vi "数据查询筛选.vi"() -> (2 "分钟小时":string(combo)="实时数据", 3 "工作类型":string(combo)="全部数据")   [LabVIEW 2016, in "斯坦道CODMn.lvlib"]
panel:
  in  "布尔":bool
  in  "数据类型 2":string(combo)="实时数据"
  in  "数据类型":string(combo)="全部数据"
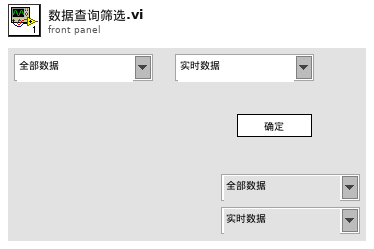
[diagram p1: front panel]
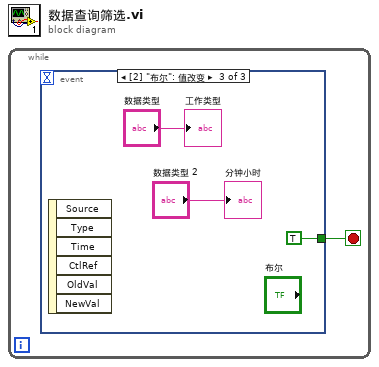
[diagram p0: block diagram]
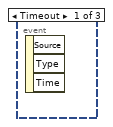
[diagram p2: hidden frame]
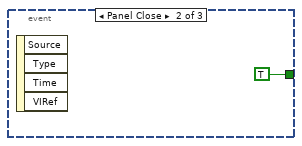
[diagram p3: hidden frame]
diagram:
  n1 = while {
    stop <- w1 stop-if-true
    n2 = event shown="[2] \"布尔\": 值改变" {
      selector: _ -> [_ _ _]
      dyn-events: _ -> [_ _ _]
      timeout: _ -> [_ _ _]
      tunnel: [_ TRUE TRUE] -> w1
      event Timeout {
        n3 = event-data() -> ()  [unwired: 1 in, 3 out]
      }
      event Panel Close {
        n4 = event-data() -> ()  [unwired: 1 in, 4 out]
      }
      event "布尔": Value Change {
        n5 = event-data() -> ()  [unwired: 1 in, 6 out]
        "工作类型" <- "数据类型"
        "分钟小时" <- "数据类型 2"
      }
    }
  }
